vi "PressureRead.vi"() -> ()   [LabVIEW 2011]
uses:
  <vilib>/LabVIEW Interface for Arduino/Type Defs/Pin Mode.ctl
  <vilib>/LabVIEW Interface for Arduino/LabVIEW Interface for Arduino.lvlib
panel:
  out "PWM Pins":u8[](array[numeric])
  in  "PWM Pin (6)":u8=5
  in  "PWM Pin (5)":u8=6
  in  "PWM Pin (3)":u8=3
  in  "Move Motor":bool
  in  "Duty Cycle":dbl min=0.0 max=255.0 step=1.0 format="%#_3g"
  out "PressureOffset":dbl
  in  "Zero":bool
  out "Waveform Chart":dbl(graph)
  out "Pressure (psi)":dbl
  in  "Analog Input Pin (0)":u8=1
  in  "ValveOpen?":bool
  in  "Valve I/O Pin":u8=2
  in  "Pin Mode":T1=enum."Output"
  in  "stop":bool
  in  "VISA resource":refnum<visa-resource-name>="COM5"
  # "Open/Close Valve"
  # "Pressure Sensor"
  # "Motor Control"
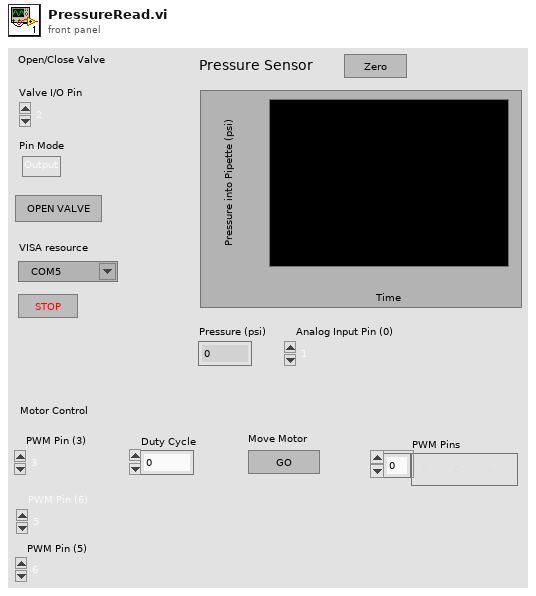
[diagram p1: front panel]
types:
  T1 = typedef "LabVIEW Interface for Arduino.lvlib/Pin Mode.ctl" = enum8{"Input", "Output"}
  T2 = typedef "LabVIEW Interface for Arduino.lvlib/Arduino Resource.ctl" = cluster{"VISA resource":refnum<visa-resource-name>, "Board Type":T3, "Connection Type":enum8{"USB / Serial"}, "Bytes Per Packet (15)":u8}
  T3 = typedef "LabVIEW Interface for Arduino.lvlib/Board Type.ctl" = enum16{"Uno", "Dimuelanove w/Atmega 328", "Mega 2560"}
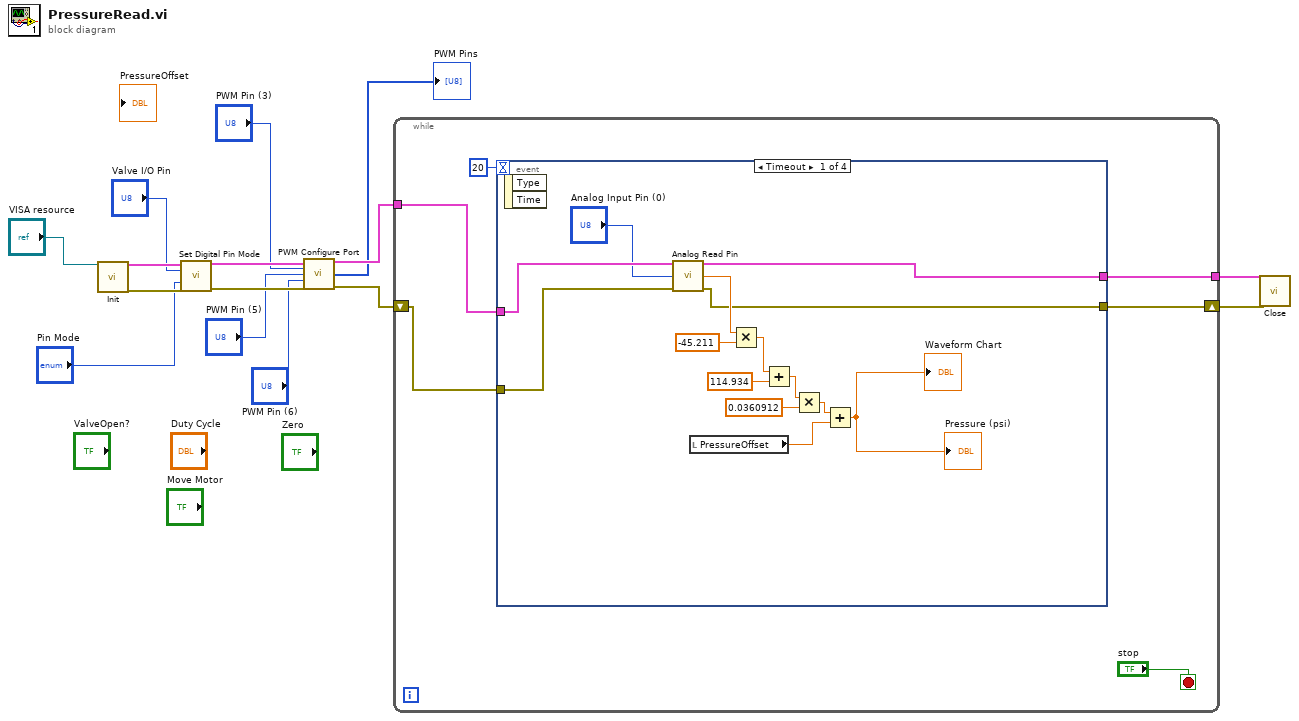
[diagram p0: block diagram]
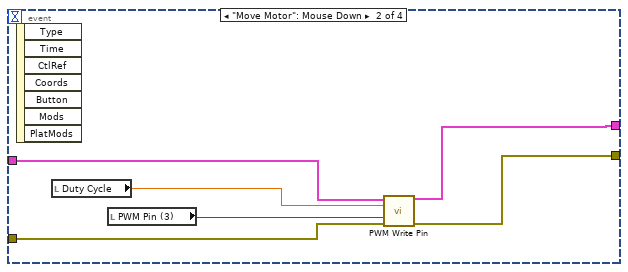
[diagram p2: hidden frame]
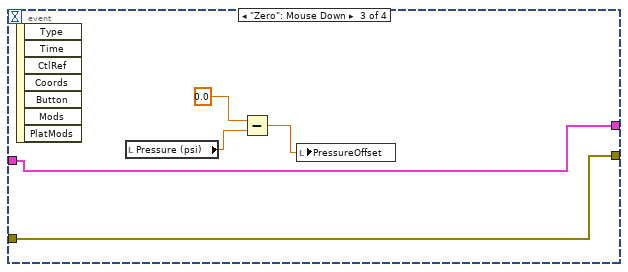
[diagram p3: hidden frame]
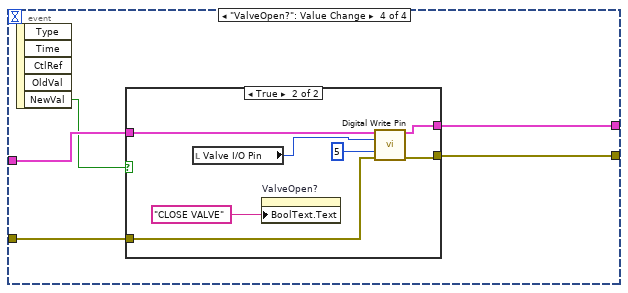
[diagram p4: hidden frame]
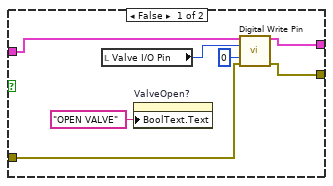
[diagram p5: hidden frame]
diagram:
  n1 = call <vilib>:"Init.vi"("VISA resource"="VISA resource") -> ("Arduino Resource"=w14:T2, "error out"=w13:errorcluster)  [unwired: 17 in]
  n2 = call <vilib>:"Set Digital Pin Mode.vi"("Arduino Resource"=w14, "Digital I/O Pin"="Valve I/O Pin", "Pin Mode (Input)"="Pin Mode", "error in"=w13) -> ("Arduino Resource"=w7:T2, "error out"=w6:errorcluster)  [unwired: 10 in]
  n3 = call <vilib>:"PWM Configure Port.vi"("Arduino Resource"=w7, "PWM Pin (3)"="PWM Pin (3)", "PWM Pin (5)"="PWM Pin (5)", "PWM Pin (6)"="PWM Pin (6)", "error in"=w6) -> ("Arduino Resource"=w9:T2, "PWM Pins"=→"PWM Pins":u8[], "error out"=w8:errorcluster)  [unwired: 8 in]
  n4 = while {
    tunnel: w9 -> [w20]
    tunnel: [w19] -> w11
    shift-right: [w17] -> w10
    shift-left: w8 -> [w18]
    stop <- "stop" stop-if-true
    n5 = event shown="[0] Timeout" {
      selector: _ -> [_ _ _ _]
      dyn-events: _ -> [_ _ _ _]
      timeout: 20 -> [_ _ _ _]
      tunnel: w20 -> [w35 w41 w43 w51]
      tunnel: w18 -> [w34 w40 w42 w49]
      tunnel: [w23 w37 w43 w48] -> w19
      tunnel: [w22 w36 w42 w47] -> w17
      event Timeout {
        n6 = event-data() -> ()  [unwired: 1 in, 2 out]
        n7 = call <vilib>:"Analog Read Pin.vi"("Arduino Resource"=w35, "Analog Input Pin (0)"="Analog Input Pin (0)", "error in"=w34) -> ("Arduino Resource"=w23:T2, "Voltage"=w32:dbl, "error out"=w22:errorcluster)  [unwired: 10 in]
        n8 = local read "PressureOffset"() -> (w25:dbl)
        n9 = Multiply(x=w32, y=-45.211) -> (x*y=w30:dbl)
        n10 = Add(x=w30, y=114.934) -> (x+y=w28:dbl)
        n11 = Multiply(x=w28, y=0.0360912) -> (x*y=w26:dbl)
        n12 = Add(x=w26, y=w25) -> (x+y=→"Pressure (psi)" →"Waveform Chart":dbl)
      }
      event "Move Motor": Mouse Down {
        n13 = event-data() -> ()  [unwired: 1 in, 7 out]
        n14 = local read "Duty Cycle"() -> (w38:dbl)
        n15 = local read "PWM Pin (3)"() -> (w39:u8)
        n16 = call <vilib>:"PWM Write Pin.vi"("Arduino Resource"=w41, "Duty Cycle (0 - 255)"=w38, "PWM Pin (3)"=w39, "error in"=w40) -> ("Arduino Resource"=w37:T2, "error out"=w36:errorcluster)  [unwired: 10 in]
      }
      event "Zero": Mouse Down {
        n17 = event-data() -> ()  [unwired: 1 in, 7 out]
        n18 = local read "Pressure (psi)"() -> (w45:dbl)
        n19 = Subtract(x=0.0, y=w45) -> (x-y=w44:dbl)
        n20 = local write "PressureOffset"(w44) -> ()
      }
      event "ValveOpen?": Value Change {
        n21 = event-data() -> ("NewVal"=w50:bool)  [unwired: 1 in, 4 out]
        n22 = case shown="True" w50 {
          tunnel: w51 -> [w58 w65]
          tunnel: w49 -> [w54 w61]
          tunnel: [w57 w60] -> w48
          tunnel: [w53 w59] -> w47
          frame False {
            n23 = local read "Valve I/O Pin"() -> (w56:u8)
            n24 = property on="ValveOpen?" class="Bool"("BoolText.Text"="OPEN VALVE" ("Caption.Text")) -> ()  [unwired: 2 in, 2 out]
            n25 = call <vilib>:"Digital Write Pin.vi"("Arduino Resource"=w58, "Digital I/O Pin (0)"=w56, "Value (0)"=u8 0, "error in"=w54) -> ("Arduino Resource"=w57:T2, "error out"=w53:errorcluster)  [unwired: 10 in]
          }
          frame True {
            n26 = local read "Valve I/O Pin"() -> (w62:u8)
            n27 = property on="ValveOpen?" class="Bool"("BoolText.Text"="CLOSE VALVE" ("Caption.Text")) -> ()  [unwired: 2 in, 2 out]
            n28 = call <vilib>:"Digital Write Pin.vi"("Arduino Resource"=w65, "Digital I/O Pin (0)"=w62, "Value (0)"=u8 5, "error in"=w61) -> ("Arduino Resource"=w60:T2, "error out"=w59:errorcluster)  [unwired: 10 in]
          }
        }
      }
    }
  }
  n29 = call <vilib>:"Close.vi"("Arduino Resource"=w11, "error in"=w10) -> ()  [unwired: 13 in, 1 out]
